vi "gpibdriver.vi"(0 "Characters to Write":string, 1 "Read":bool, 2 "Write":bool, 3 "GPIB\nAddress":string="1", 4 "timeout":u32=5000, 6 "# bytes\nto read":i32=200 format="%0.0f") -> (5 "Characters Read":string)   [LabVIEW 2015]
doc: "A device connected to a GPIB bus can be written to or be read from using this VI. Select the GPIB address of the device, choose Read or Write or both, type in the characters to be written, and run the VI. If you choose both Read and Write, the VI will write to the device first, then read from the device. Before using this VI you should initialize the GPIB address according to the device's specifications with the \"GPIB Initialization\" function."
panel:
  out "Write Status":string
  out "Read Status":string
  # "Select  the GPIB address of the device, choose Read or Write or both, type in the characters to be written, and run the VI. If you choose both Read and Write, the VI will write to the device first, then read from the device.  Before using this VI, you should consider initializing the bus with the \"GPIB Initialization\" function."
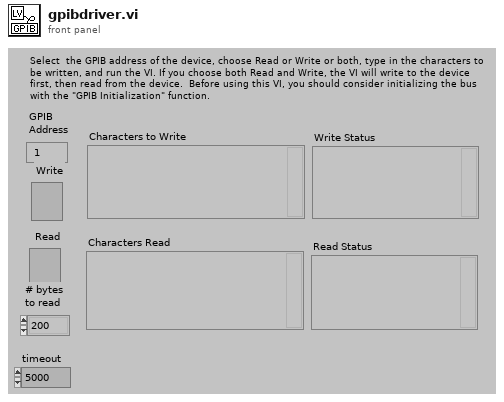
[diagram p1: front panel]
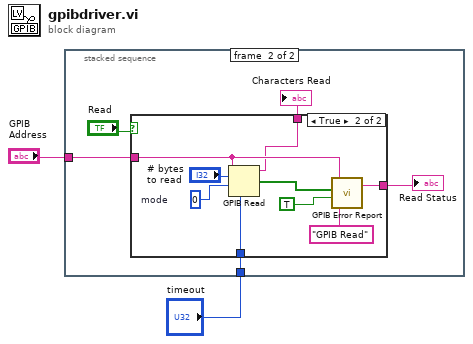
[diagram p0: block diagram]
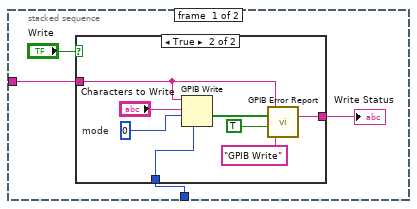
[diagram p2: hidden frame]
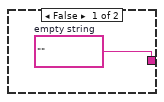
[diagram p3: hidden frame]
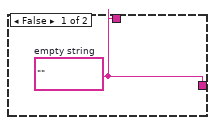
[diagram p4: hidden frame]
diagram:
  n1 = stacked-sequence {
    tunnel: "GPIB\nAddress" -> [w6 w20]
    tunnel: "timeout" -> [w3 w16]
    frame #0 {
      n2 = case shown="True" "Write" {
        tunnel: [w7 w9] -> w4
        tunnel: w6 -> [_ w13]
        tunnel: w3 -> [_ w8]
        frame False {
          w7 = ""  # empty string
        }
        frame True {
          w15 = 0  # mode
          n3 = GPIB Write(0:w13, 1:"Characters to Write", 2:w15, 4:w8) -> (5:w12:bool[])  [unwired: 1 in, 1 out]
          n4 = call "GPIB Error Report.vi"("Function"="GPIB Write", "Dialog?(F)"=TRUE, "Status"=w12, "Address String"=w13) -> ("Status String"=w9:string)  [unwired: 1 out]
        }
      }
      "Write Status" <- w4
    }
    frame #1 {
      n5 = case shown="True" "Read" {
        tunnel: [w21 w24] -> w17
        tunnel: [w21 w25] -> w18
        tunnel: w20 -> [_ w29]
        tunnel: w16 -> [_ w22]
        frame False {
          w21 = ""  # empty string
        }
        frame True {
          w30 = 0  # mode
          n6 = GPIB Read(0:w29, 1:"# bytes\nto read", 2:w30, 4:w22) -> (5:w24:string, 6:w23:bool[])  [unwired: 1 in, 1 out]
          n7 = call "GPIB Error Report.vi"("Function"="GPIB Read", "Dialog?(F)"=TRUE, "Status"=w23, "Address String"=w29) -> ("Status String"=w25:string)  [unwired: 1 out]
        }
      }
      "Characters Read" <- w17
      "Read Status" <- w18
    }
  }
